vi "MeasureInLoop.vi"() -> ()   [LabVIEW 2015]
uses:
  Anemometry Sub Vis/Controls/MeasureInLoop.ctl
  Anemometry Sub Vis/File/Setup_Filetype.ctl
  Anemometry Sub Vis/Controls/Post_Process.ctl
  Anemometry Sub Vis/Controls/Save_Data.ctl
  Anemometry Sub Vis/Controls/Setup.ctl
  Anemometry Sub Vis/Globals/Meas_global.vi
  Anemometry Sub Vis/Globals/Trav_pos_global.vi
panel:
  in  "Tab Control":enum32{"Setup", "MeasGraph2", "Debug"}(tab)
  in  "Setup:":string(combo)="Current_Setup.xls"
  in  "File by:":enum16{"Day", "Week", "Month"}(ring)=enum."Week"
  in  "Measure (seconds)":dbl=60.0
  in  "Wait (minutes)":dbl=15.0
  out "MeasurementsTaken:":i32
  out "XY Graph":cluster{"X array":dbl[], "Y array":dbl[]}[](graph)
  out "CurrentFilename":string
  out "Task":T1=enum."Initialise"
  in  "Stop Button":bool
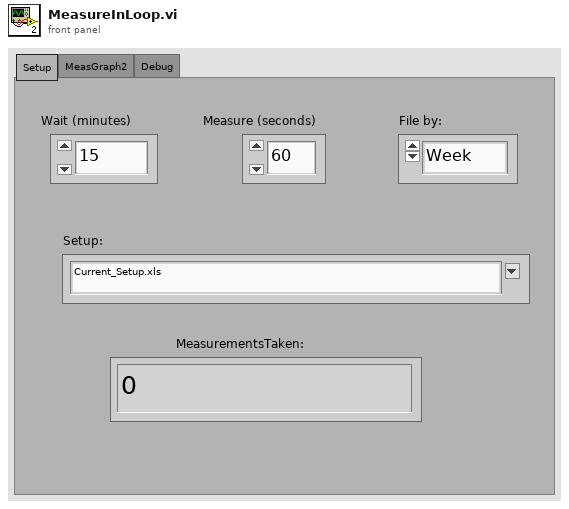
[diagram p1: front panel]
types:
  T1 = typedef "MeasureInLoop.ctl" = enum16{"RunHub", "Initialise", "Take Measurement", "Start Waiting", "End"}
  T2 = typedef "Setup.ctl" = enum16{"Run Program", "Show Setup", "Save Current Setup", "Setup Front Panel"}
  T3 = typedef "Save_Data.ctl" = enum16{"Save No Data", "Save Data"}
  T4 = typedef "Post_Process.ctl" = enum16{"Take New Data", "Post Process Raw Data File"}
  T5 = typedef "Setup_Filetype.ctl" = enum16{"Measurement Setups", "Calibration Setups", "General", "Results File Plotter Setups", "Speed Calib Tweaks"}
  T6 = typedef "Traverse_cluster.ctl" = cluster{"Start X":sgl, "Start Y":sgl, "Start Z":sgl, "End X":sgl, "End Y":sgl, "End Z":sgl, "No. of pts.":i32, "Spacing":T7, "Filename":path, "Tunnel Speed":dbl, "Averaging time (min)":dbl, "Extra Commands":string, "Carrier_1 Q (l/min)":dbl, "Carrier_2 Q (l/min)":dbl, "Trace Gas Concentration (%)":dbl, "Specific Arguments":string, "Comments":string, "Row No":i32, "Row Type Selector":T8, "Completion time":string, "Row Duration (mins)":dbl, "No. of Valid pts.":i32, "Meas Setup File":string}
  T7 = typedef "Spacing.ctl" = enum16{"Linear", "Log", "Gauss", "Specified", "N/A"}
  T8 = typedef "Multi_run_mode.ctl" = enum16{"Move Traverse Only", "Set Tunnel Speed Only", "Set Source Only", "Set Measurement Conditions", "Single Measurement", "Vertical Profile", "Lateral Profile", "Longitudinal Profile", "Explore Volume", "Multi-Axis Profile", "Auto Calibrate", "Meas Fast FID Bkgnd", "Check Beam Power", "Scanning Valve Measurement", "Run VI Named:", "Set ADAM Ch", "Wait (minutes)", "Send Message", "Synchronize With:", "Fall Back to this Row", "Turn Off Row Repeating", "Blank Row", "Traverse 3D Volume"}
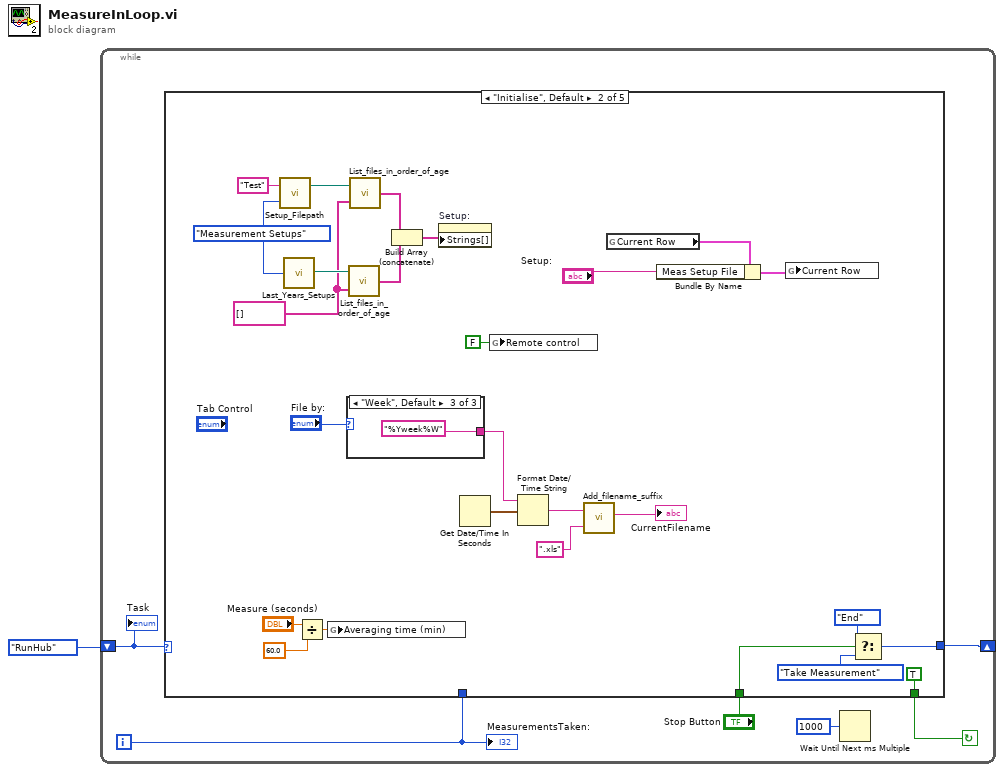
[diagram p0: block diagram]
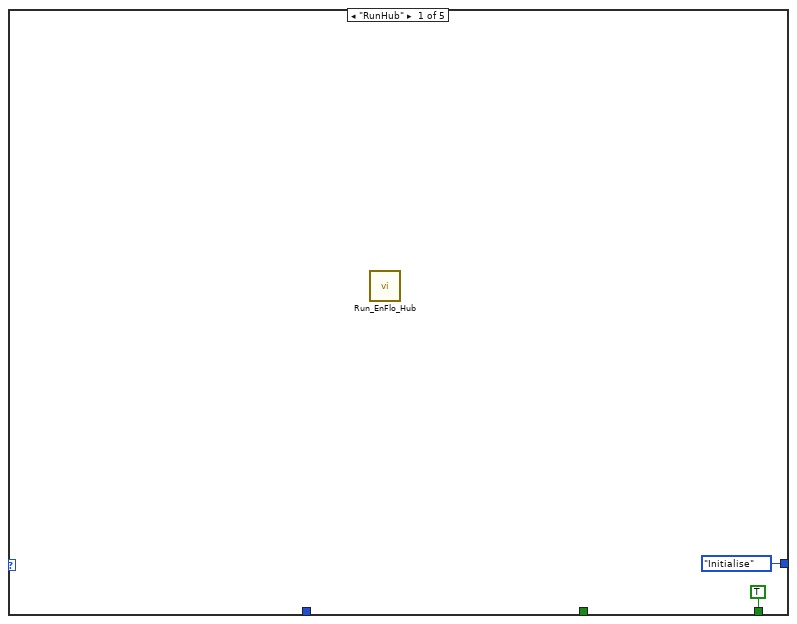
[diagram p2: hidden frame]
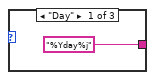
[diagram p3: hidden frame]
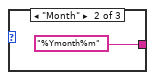
[diagram p4: hidden frame]
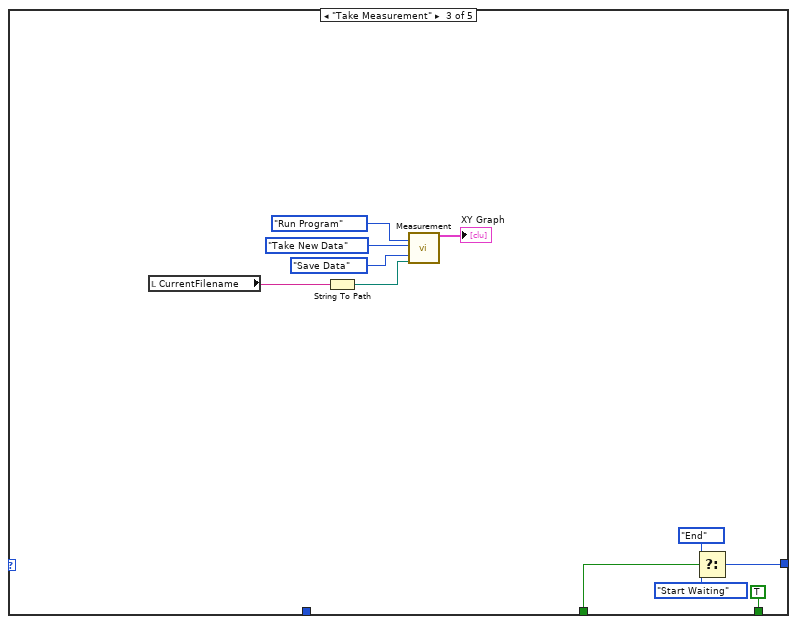
[diagram p5: hidden frame]
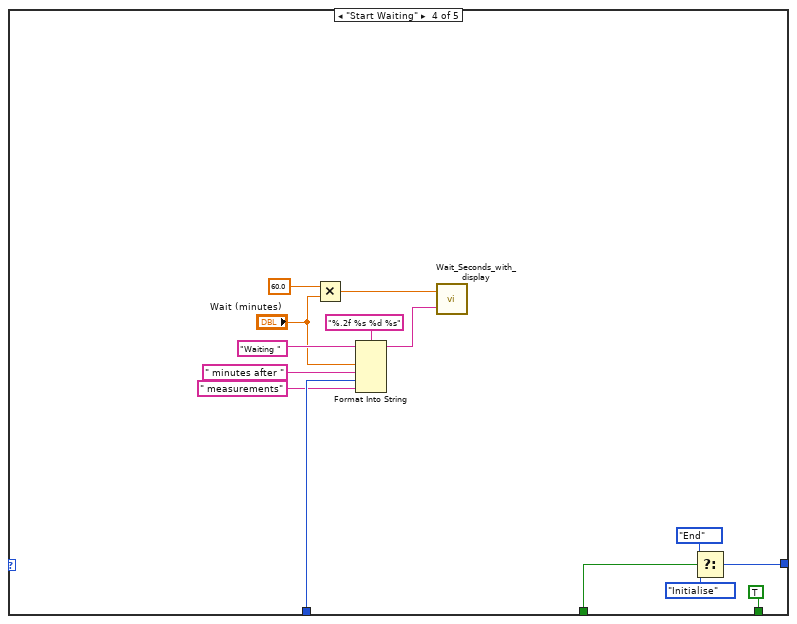
[diagram p6: hidden frame]
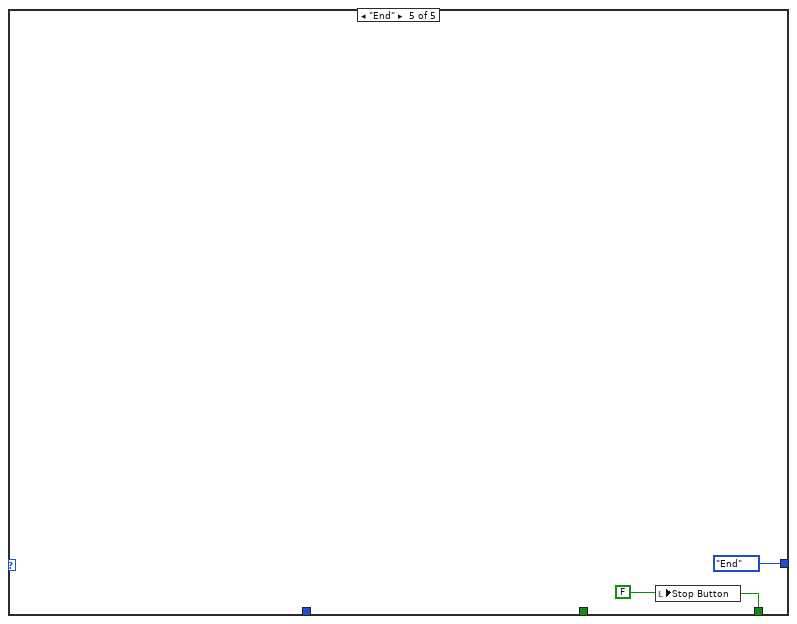
[diagram p7: hidden frame]
diagram:
  n1 = while {
    shift-right: [w6] -> _
    shift-left: MeasureInLoop."RunHub" ("Task") -> [w4]
    i -> [w7]
    stop <- w5 continue-if-true
    n2 = case shown="\"Initialise\", Default" w4 {
      tunnel: w7 -> [_ _ _ w57 _]
      tunnel: [MeasureInLoop."Initialise" ("Task") w12 w42 w52 MeasureInLoop."End" ("Task")] -> w6
      tunnel: [TRUE ("Stop Button") TRUE ("Stop Button") TRUE ("Stop Button") TRUE ("Stop Button") w64] -> w5
      tunnel: "Stop Button" -> [_ w10 w39 w50 _]
      frame "RunHub" {
        n3 = call "Run_EnFlo_Hub.vi"() -> ()  [unwired: 1 in, 7 out]
      }
      frame "Initialise", Default {
        w25 = Setup_Filetype."Measurement Setups" ("Setup File Type")
        w20 = string[] [] ("file names")
        n4 = call "Setup_Filepath.vi"("Setup File Type"=w25, "Filename in"="Test") -> ("Directory"=w24:path)  [unwired: 1 out]
        n5 = call "Last_Years_Setups.vi"("Setup File Type"=w25) -> ("Directory"=w26:path)
        n6 = Divide(x="Measure (seconds)", y=60.0 ("x")) -> (x/y=w27:dbl)
        n7 = global write "Meas_global.vi" "Averaging time (min)"(w27) -> ()
        n8 = case shown="\"Week\", Default" "File by:" {
          tunnel: ["%Yday%j" ("FilenameFormatter") "%Ymonth%m" ("FilenameFormatter") "%Yweek%W" ("FilenameFormatter")] -> w33
          frame "Day" {
          }
          frame "Month" {
          }
          frame "Week", Default {
          }
        }
        n9 = call "List_files_in_order_of_age.vi"("Files to Hide"=w20, "Folder"=w26) -> ("file names"=w22:string[])
        n10 = call "List_files_in_order_of_age.vi"("Files to Hide"=w20, "Folder"=w24) -> ("file names"=w23:string[])
        n11 = Build Array (concatenate)(w23, w22) -> (w19:string[])
        n12 = property on="Setup:" class="CmbBox"("Strings[]"=w19) -> ()  [unwired: 2 in, 2 out]
        n13 = Get Date/Time In Seconds() -> (seconds since 1Jan1904=w35:timestamp)
        n14 = global write "Meas_global.vi" "Remote control"(FALSE ("Remote control")) -> ()
        n15 = Format Date/Time String(time format string (%c)=w33, seconds (now)=w35) -> (date/time string=w32:string)  [unwired: 1 in]
        n16 = call "Add_filename_suffix.vi"("Filename"=w32, "Suffix to add"=".xls") -> ("Filename out"=→"CurrentFilename":string)  [unwired: 3 out]
        n17 = global read "Trav_pos_global.vi" "Current Row"() -> (w17:T6)
        n18 = Bundle By Name(cluster=w17, "Meas Setup File"="Setup:") -> (w16:T6)
        n19 = global write "Trav_pos_global.vi" "Current Row"(w16) -> ()
        n20 = Select(t=MeasureInLoop."End" ("Task"), s=w10, f=MeasureInLoop."Take Measurement" ("Task")) -> (s? t:f=w12:T1)
      }
      frame "Take Measurement" {
        n21 = local read "CurrentFilename"() -> (w44:string)
        n22 = String To Path(string=w44) -> (path=w49:path)
        n23 = call "Measurement.vi"("setup"=Setup."Run Program", "Post Process"=Post_Process."Take New Data", "File"=Save_Data."Save Data", "Results file"=w49) -> ("2nd plot"=→"XY Graph":cluster{"X array":dbl[], "Y array":dbl[]}[])  [unwired: 3 in, 12 out]
        n24 = Select(t=MeasureInLoop."End" ("Task"), s=w39, f=MeasureInLoop."Start Waiting" ("Task")) -> (s? t:f=w42:T1)
      }
      frame "Start Waiting" {
        n25 = Multiply(x=60.0 ("value"), y="Wait (minutes)") -> (x*y=w63:dbl)
        n26 = Format Into String(format string="%.2f %s %d %s", initial string="Waiting " ("Message"), "Wait (minutes)", " minutes after " ("Message"), w57, " measurements" ("Message")) -> (resulting string=w60:string)  [unwired: 1 in, 1 out]
        n27 = call "Wait_Seconds_with_display.vi"("Message"=w60, "Seconds to wait"=w63) -> ()  [unwired: 1 in, 1 out]
        n28 = Select(t=MeasureInLoop."End" ("Task"), s=w50, f=MeasureInLoop."Initialise" ("Task")) -> (s? t:f=w52:T1)
      }
      frame "End" {
        w64 = FALSE ("Stop Button")
        n29 = local write "Stop Button"(w64) -> ()
      }
    }
    n30 = Wait Until Next ms Multiple(millisecond multiple=u32 1000) -> ()  [unwired: 1 out]
    "MeasurementsTaken:" <- w7
    "Task" <- w4
  }
